vi "connection.vi"(2 "error out":errorcluster, 3 "VISA resource name":refnum<visa-resource-name>) -> (0 "error out 2":errorcluster, 1 "VISA resource name 2":refnum<visa-resource-name>)   [LabVIEW 2017]
panel:
  out "Array":string[](array[string])
  out "millisecond timer value":u32[](array[numeric]) format="%.2f"
  out "read buffer":string[](array[string])
  out "Boolean":bool
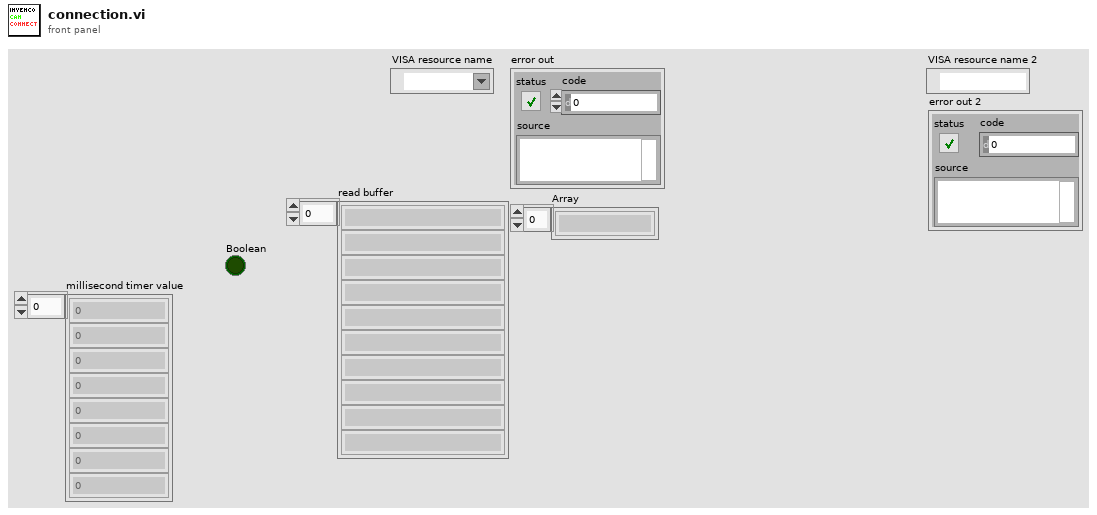
[diagram p1: front panel]
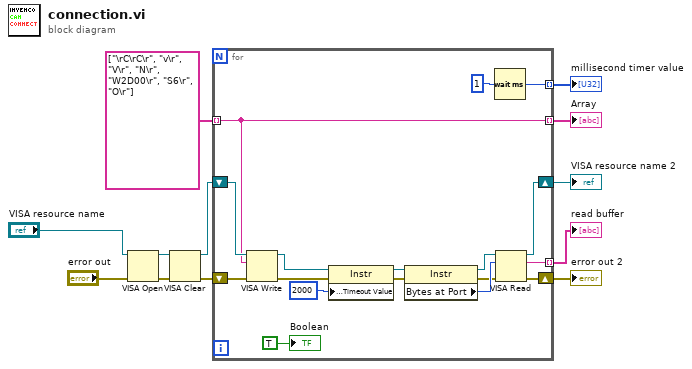
[diagram p0: block diagram]
diagram:
  n1 = VISA Open(error in (no error)="error out", VISA resource name="VISA resource name") -> (VISA resource name=w6:refnum<visa-resource-name>, error out=w5:errorcluster)  [unwired: 3 in]
  n2 = VISA Clear(VISA resource name=w6, error in (no error)=w5) -> (VISA resource name out=w1:refnum<visa-resource-name>, error out=w3:errorcluster)
  n3 = for {
    tunnel: string[] ["\rC\rC\r", "v\r", "V\r", "N\r", "W2D00\r", "S6\r", "O\r"] -> [w13] mode=indexing
    shift-right: [w27] -> w9
    shift-left: w1 -> [w29]
    shift-right: [w26] -> w8
    shift-left: w3 -> [w28]
    tunnel: [w16] -> w12 mode=indexing
    tunnel: [w15] -> w11 mode=indexing
    tunnel: [w13] -> w7 mode=indexing
    n4 = VISA Write(VISA resource name=w29, write buffer=w13, error in (no error)=w28) -> (VISA resource name out=w21:refnum<visa-resource-name>, error out=w20:errorcluster)  [unwired: 1 out]
    n5 = property class="Instr"(reference=w21, error in=w20, "General Settings:Timeout Value"=u32 2000) -> (reference out=w18:refnum<visa-resource-name>, error out=w19:errorcluster)
    n6 = property class="Instr"(reference=w18, error in=w19) -> (reference out=w24:refnum<visa-resource-name>, error out=w23:errorcluster, "Bytes at Port"=w25:u32)
    n7 = Wait (ms)(milliseconds to wait=u32 1 ("millisecond multiple")) -> (millisecond timer value=w15:u32)
    n8 = VISA Read(VISA resource name=w24, byte count=w25, error in (no error)=w23) -> (VISA resource name out=w27:refnum<visa-resource-name>, read buffer=w16:string, error out=w26:errorcluster)  [unwired: 1 out]
    "Boolean" <- TRUE
  }
  "read buffer" <- w12
  "millisecond timer value" <- w11
  "VISA resource name 2" <- w9
  "error out 2" <- w8
  "Array" <- w7
